vi "Zoom Manager.vi"(7 "Command":enum16{"Zoom IN", "Zoom OUT", "Fit"}(ring), 8 "error in (no error)":errorcluster, 10 "Image":refnum<vi>, 11 "Zoom Cluster":refnum<vi>) -> (0 "error out":errorcluster)   [LabVIEW 2024]
uses:
  Buttons/Zoom Out.ctl
  Buttons/Zoom Inn.ctl
  Buttons/Zoom Fit.ctl
  <vilib>/Utility/miscctls.llb/LVPointTypeDef.ctl
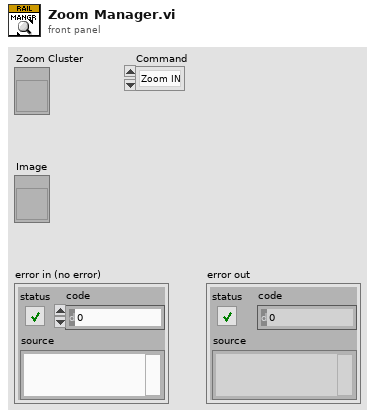
[diagram p1: front panel]
types:
  T1 = typedef "Zoom Out.ctl" = bool
  T2 = typedef "Zoom Inn.ctl" = bool
  T3 = typedef "Zoom Fit.ctl" = bool
  T4 = cluster{"Zoom Out":T1, "Zoom In":T2, "Zoom Fit":T3}
  T5 = typedef "LVPointTypeDef.ctl" = cluster{"Horizontal":i16, "Vertical":i16}
  T6 = typedef "LVBoundsTypeDef.ctl" = cluster{"Width":u32, "Height":u32}
  T7 = typedef "imagedata.ctl" = cluster{"image type":i32, "image depth":i32, "image":u8[], "mask":u8[], "colors":u32[], "Rectangle":cluster{"left":i16, "top":i16, "right":i16, "bottom":i16}}
  T8 = cluster{"left":i16, "top":i16, "right":i16, "bottom":i16}
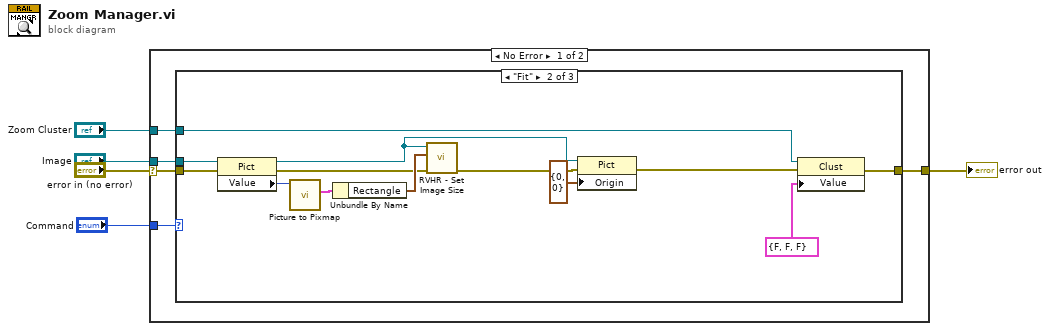
[diagram p0: block diagram]
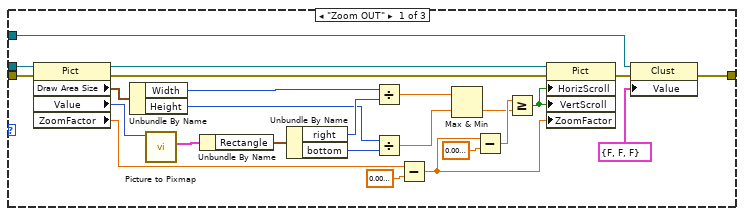
[diagram p2: hidden frame]
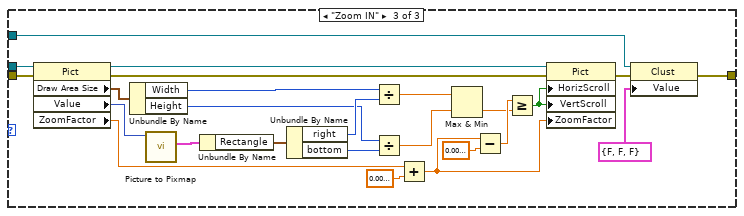
[diagram p3: hidden frame]
diagram:
  n1 = case shown="No Error" "error in (no error)" {
    selector: "error in (no error)" -> [w7 w74]
    tunnel: "Zoom Cluster" -> [w10 _]
    tunnel: "Image" -> [w9 _]
    tunnel: [w8 w74] -> w3
    tunnel: "Command" -> [w6 _]
    frame No Error {
      n2 = case shown="\"Fit\"" w6 {
        tunnel: w10 -> [w34 w47 w72]
        tunnel: w9 -> [w13 w41 w51]
        tunnel: [w12 w46 w50] -> w8
        tunnel: w7 -> [w11 w42 w49]
        frame "Zoom OUT" {
          n3 = property class="Pict"(reference=w13, error in=w11) -> (reference out=w14:refnum<vi>, error out=w15:errorcluster, "Draw Area Size"=w27:T6, "Value"=w18:picture, "ZoomFactor"=w16:sgl)
          n4 = Unbundle By Name(w27) -> ("Width"=w21:u32, "Height"=w22:u32)
          n5 = call <vilib>:"Picture to Pixmap.vi"("picture"=w18) -> ("image data"=w19:T7)  [unwired: 9 in, 1 out]
          n6 = Unbundle By Name(w19) -> ("Rectangle"=w28:T8)
          n7 = Unbundle By Name(w28) -> ("right"=w25:i16, "bottom"=w26:i16)
          n8 = Divide(x=w21, y=w25) -> (x/y=w23:dbl)
          n9 = Divide(x=w22, y=w26) -> (x/y=w24:dbl)
          n10 = Subtract(x=w16, y=sgl 0.01) -> (x-y=w31:sgl)
          n11 = Max & Min(x=w23, y=w24) -> (min(x,y)=w20:dbl)  [unwired: 1 out]
          n12 = Subtract(x=w31, y=sgl 0.01) -> (x-y=w32:sgl)
          n13 = Greater Or Equal?(x=w32, y=w20) -> (x >= y?=w29:bool)
          n14 = property class="Pict"(reference=w14, error in=w15, "HorizScroll"=w29, "VertScroll"=w29, "ZoomFactor"=w31) -> (error out=w33:errorcluster)  [unwired: 1 out]
          n15 = property class="Clust"(reference=w34, error in=w33, "Value"=T4 {"Zoom Out"=FALSE, "Zoom In"=FALSE, "Zoom Fit"=FALSE} ("Zoom Toolbar L")) -> (error out=w12:errorcluster)  [unwired: 1 out]
        }
        frame "Fit" {
          n16 = property class="Pict"(reference=w41, error in=w42) -> (reference out=w37:refnum<vi>, error out=w44:errorcluster, "Value"=w43:picture)
          n17 = call <vilib>:"Picture to Pixmap.vi"("picture"=w43) -> ("image data"=w40:T7)  [unwired: 9 in, 1 out]
          n18 = Unbundle By Name(w40) -> ("Rectangle"=w45:T8)
          n19 = call "RVHR - Set Image Size.vi"("error in (no error)"=w44, "Rectangle"=w45, "Image_L"=w37) -> ("error out"=w39:errorcluster)  [unwired: 8 in]
          n20 = property class="Pict"(reference=w37, error in=w39, "Origin"=T5 {"Horizontal"=0, "Vertical"=0}) -> (error out=w38:errorcluster)  [unwired: 1 out]
          n21 = property class="Clust"(reference=w47, error in=w38, "Value"=T4 {"Zoom Out"=FALSE, "Zoom In"=FALSE, "Zoom Fit"=FALSE} ("Zoom Toolbar L")) -> (error out=w46:errorcluster)  [unwired: 1 out]
        }
        frame "Zoom IN" {
          n22 = property class="Pict"(reference=w51, error in=w49) -> (reference out=w52:refnum<vi>, error out=w53:errorcluster, "Draw Area Size"=w65:T6, "Value"=w56:picture, "ZoomFactor"=w54:sgl)
          n23 = Unbundle By Name(w65) -> ("Width"=w59:u32, "Height"=w60:u32)
          n24 = call <vilib>:"Picture to Pixmap.vi"("picture"=w56) -> ("image data"=w57:T7)  [unwired: 9 in, 1 out]
          n25 = Unbundle By Name(w57) -> ("Rectangle"=w66:T8)
          n26 = Unbundle By Name(w66) -> ("right"=w63:i16, "bottom"=w64:i16)
          n27 = Divide(x=w59, y=w63) -> (x/y=w61:dbl)
          n28 = Divide(x=w60, y=w64) -> (x/y=w62:dbl)
          n29 = Add(x=w54, y=sgl 0.01) -> (x+y=w69:sgl)
          n30 = Max & Min(x=w61, y=w62) -> (min(x,y)=w58:dbl)  [unwired: 1 out]
          n31 = Subtract(x=w69, y=sgl 0.01) -> (x-y=w70:sgl)
          n32 = Greater Or Equal?(x=w70, y=w58) -> (x >= y?=w67:bool)
          n33 = property class="Pict"(reference=w52, error in=w53, "HorizScroll"=w67, "VertScroll"=w67, "ZoomFactor"=w69) -> (error out=w71:errorcluster)  [unwired: 1 out]
          n34 = property class="Clust"(reference=w72, error in=w71, "Value"=T4 {"Zoom Out"=FALSE, "Zoom In"=FALSE, "Zoom Fit"=FALSE} ("Zoom Toolbar L")) -> (error out=w50:errorcluster)  [unwired: 1 out]
        }
      }
    }
    frame Error {
    }
  }
  "error out" <- w3
